vi "Move and Hide Input Items.vi"(8 "error in (no error)":errorcluster, 10 "Name":refnum<vi>, 11 "Value":refnum<vi>) -> (0 "error out":errorcluster)   [LabVIEW 2013, in "CANopen Workspace Objects.lvlib"]
uses:
  CANopen Workspace Objects.lvlib
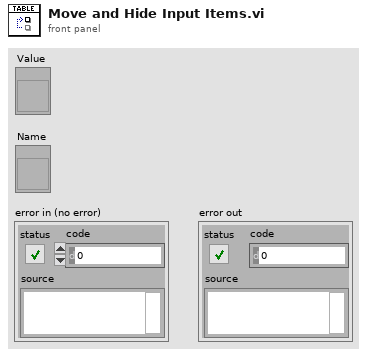
[diagram p1: front panel]
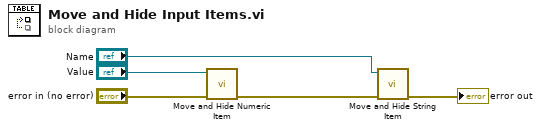
[diagram p0: block diagram]
diagram:
  n1 = call "Move and Hide Numeric Item.vi"("error in (no error)"="error in (no error)", "Digital in"="Value") -> ("error out"=w3:errorcluster)  [unwired: 9 in]
  n2 = call "Move and Hide String Item.vi"("error in (no error)"=w3, "String in"="Name") -> ("error out"=→"error out":errorcluster)  [unwired: 9 in]
